vi "Is Subscribed.vi"(8 "error in (no error)":errorcluster, 10 "Topic":string, 11 "WAMP Client in":refnum<class "WAMP Client.lvclass">) -> (0 "error out":errorcluster, 1 "SubscriptionDetailsParent out":refnum<class "SubscriptionDetailsParent.lvclass">, 2 "Found?":bool, 3 "WAMP Client out":refnum<class "WAMP Client.lvclass">)   [LabVIEW 2020, in "wamplv.lvlib" / "WAMP Client.lvclass"]
uses:
  WAMP Client.lvclass
  WAMP Client.lvclass/WAMP Client.ctl
  Private/Message loop classes/Subscription details/SubscriptionDetailsParent/SubscriptionDetailsParent.lvclass
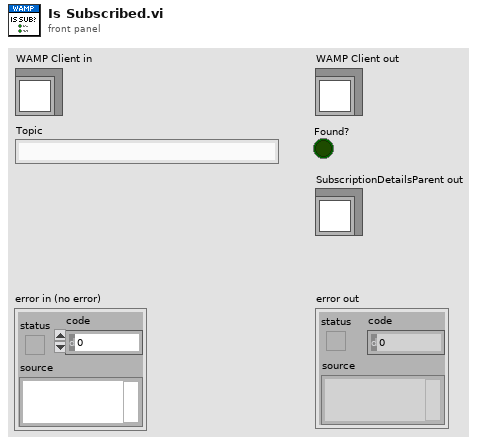
[diagram p1: front panel]
types:
  T1 = typedef "wamplv.lvlib/Message Loop Data.ctl" = cluster{"Last Request ID":u64, "Register Requests":map{u64, T2}, "Publish Requests":T3, "Endpoints Map":map{u64, T4}, "Call Requests":T5, "Subscription Requests":T6, "Subscriptions":T7, "Unsubscribe Requests":T8, "Random Request IDs":u64[], "Unregister requests map":T10}
  T2 = typedef "wamplv.lvlib/REGISTER Request Data.ctl" = cluster{"Procedure URI":string, "Options":string, "REGISTER result notifier":refnum<notifier>}
  T3 = typedef "wamplv.lvlib/Publish Requests Map.ctl" = map{u64, refnum<class "IPublish.lvclass">}
  T4 = typedef "wamplv.lvlib/Endpoint Data.ctl" = cluster{"Procedure URI":string}
  T5 = typedef "wamplv.lvlib/CALL Request Map.ctl" = map{u64, refnum<class "ICallRequest.lvclass">}
  T6 = typedef "wamplv.lvlib/SUBSCRIBE Requests Map.ctl" = map{u64, refnum<class "ISubscribe.lvclass">}
  T7 = typedef "wamplv.lvlib/Subscriptions Map.ctl" = map{u64, refnum<class "SubscriptionDetailsParent.lvclass">}
  T8 = typedef "wamplv.lvlib/Unsubscribe Requests Map.ctl" = map{u64, T9}
  T9 = typedef "wamplv.lvlib/UNSUBSCRIBE Request Data.ctl" = cluster{"Topic":string, "Unsubscrube result notifier":refnum<notifier>, "Options":string}
  T10 = typedef "wamplv.lvlib/Unregister requests map.ctl" = map{u64, T11}
  T11 = typedef "wamplv.lvlib/Unregister request.ctl" = cluster{"URI":string, "Unregister result notifier":refnum<notifier>, "Options":string}
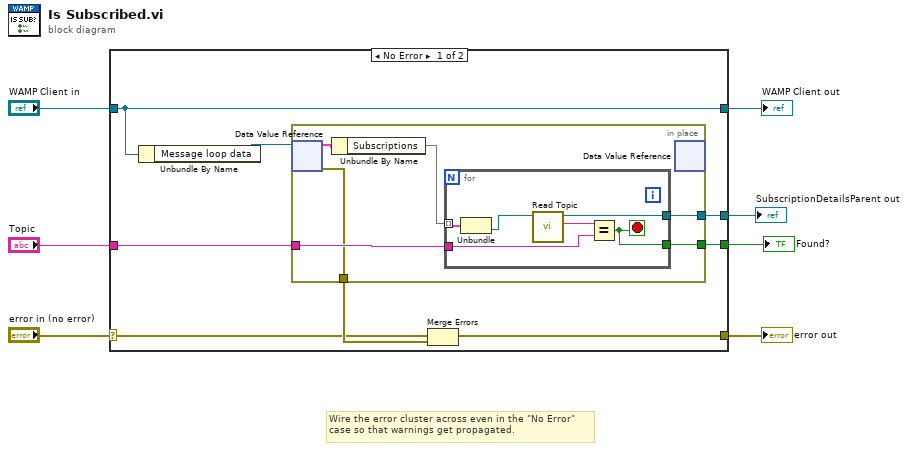
[diagram p0: block diagram]
diagram:
  # "Wire the error cluster across even in the \"No Error\"\ncase so that warnings get propagated."
  n1 = case shown="No Error" "error in (no error)" {
    selector: "error in (no error)" -> [w10 w29]
    tunnel: [w9 w29] -> w6
    tunnel: [w15 w28] -> w4
    tunnel: "WAMP Client in" -> [w15 w28]
    tunnel: "Topic" -> [w13 _]
    tunnel: [w12 _] -> w2
    tunnel: [w8 _] -> w1
    frame No Error {
      n2 = Unbundle By Name(w15) -> ("Message loop data"=w14:refnum<data-value>)
      n3 = in-place {
        in-place-border: w13 -> [w19]
        in-place-border: [w18] -> w12
        in-place-border: [w17] -> w11
        in-place-border: [w16] -> w8
        n4 = in-place-dvr #1(w14) -> (w21:T1, w17:errorcluster)
        n5 = Unbundle By Name(w21) -> ("Subscriptions"=w20:T7)
        n6 = for {
          tunnel: w20 -> [w27] mode=indexing
          tunnel: w19 -> [w26]
          tunnel: [w25] -> w18
          tunnel: [w22] -> w16
          stop <- w25 stop-if-true
          n7 = Unbundle(w27) -> ("Subscription Details"=w24:refnum<class "SubscriptionDetailsParent.lvclass">)  [unwired: 1 out]
          n8 = call "Read Topic.vi"("SubscriptionDetailsParent in"=w24) -> ("Topic"=w23:string, "SubscriptionDetailsParent out"=w22:refnum<class "SubscriptionDetailsParent.lvclass">)  [unwired: 8 in, 1 out]
          n9 = Equal?(x=w23, y=w26) -> (x = y?=w25:bool)
        }
        n10 = in-place-dvr #1() -> ()  [unwired: 1 in, 2 out]
      }
      n11 = Merge Errors(w10, w11) -> (w9:errorcluster)
    }
    frame Error {
    }
  }
  "error out" <- w6
  "WAMP Client out" <- w4
  "Found?" <- w2
  "SubscriptionDetailsParent out" <- w1
